vi "Close TDMS File.vi"(8 "Error In":errorcluster, 11 "TDMS Reference In":refnum<k34>) -> (0 "Error Out":errorcluster)   [LabVIEW 2014]
doc: "Close the reference to the specified TDMS file."
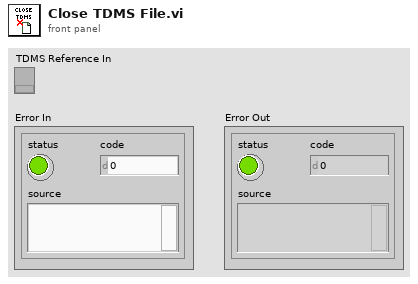
[diagram p1: front panel]
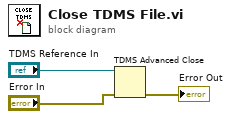
[diagram p0: block diagram]
diagram:
  n1 = TDMS Advanced Close(8:"Error In", 11:"TDMS Reference In") -> (0:→"Error Out":errorcluster)  [unwired: 2 in, 1 out]
